vi "Reformat.vi"(5 "Pretty Print?":bool, 7 "error in (no error)":errorcluster, 8 "Offset":i32, 10 "JSON":string) -> (0 "error out":errorcluster, 1 "Offset after":i32, 3 "<JSON>":string)   [LabVIEW 2015, in "JSONtext.lvlib"]
doc: "Reformat a JSON Value, either packed with all unneeded whitespace removed, or \"pretty printed\" with extra whitespace and new lines to make the JSON more human readable. This will also searve to validate the JSON."
uses:
  JSONtext.lvlib
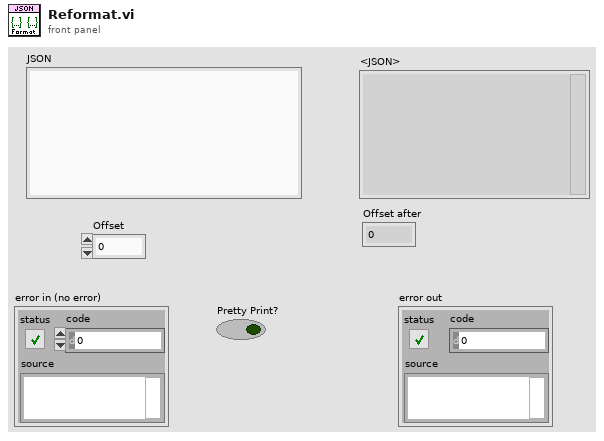
[diagram p1: front panel]
types:
  T1 = typedef "JSONtext.lvlib/Parsing State.ctl" = enum16{"Parser Error", "Object", "Array", "String", "Number/Other", "Leading Whitespace", "Object end", "Array end", "Value end"}
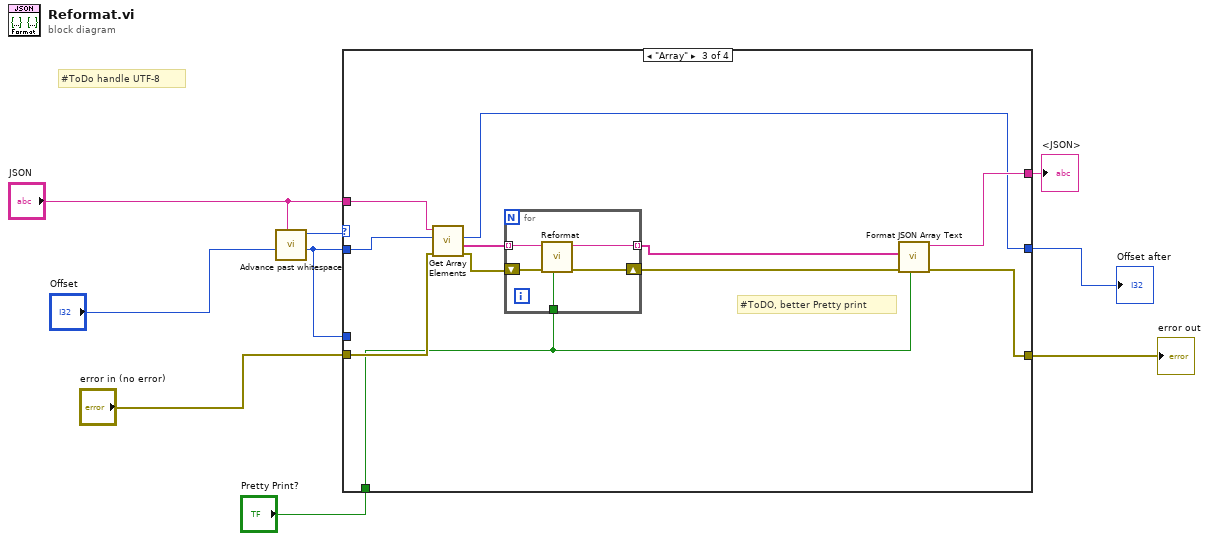
[diagram p0: block diagram]
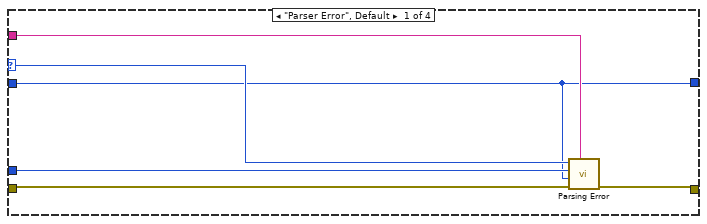
[diagram p2: hidden frame]
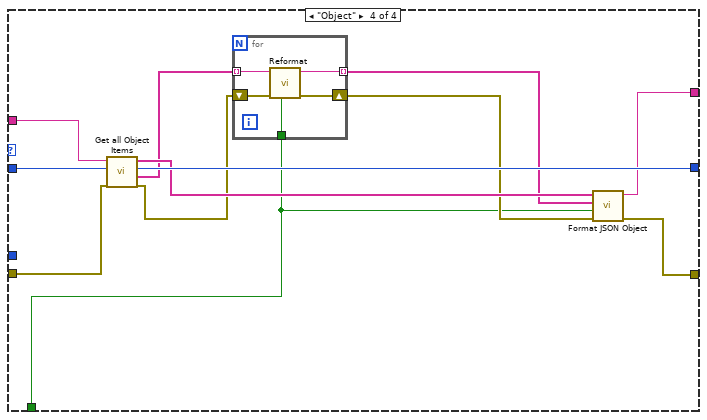
[diagram p4: hidden frame]
diagram:
  # "#ToDo handle UTF-8"
  n1 = call "Advance past whitespace.vi"("JSON"="JSON", "Offset"="Offset") -> ("Offset of first non-whitespace"=w2:i32, "Parser State"=w8:T1)  [unwired: 8 in]
  n2 = case shown="\"Array\"" w8 {
    selector: w8 -> [w13 _ _ _]
    tunnel: "JSON" -> [w11 w18 w29 w43]
    tunnel: w2 -> [w10 w16 w28 w46]
    tunnel: [w10 w16 w22 w45] -> w7
    tunnel: [_ w18 w26 w42] -> w5
    tunnel: [w15 w17 w24 w37] -> w4
    tunnel: "error in (no error)" -> [w14 w17 w23 w36]
    tunnel: w2 -> [w12 _ _ _]
    tunnel: "Pretty Print?" -> [_ _ w21 w35]
    frame "Parser Error", Default {
      n3 = call "Parsing Error.vi"("JSON"=w11, "error in (no error)"=w14, "Offset past match"=w10, "Value start"=w12, "State"=w13) -> ("error out"=w15:errorcluster)  [unwired: 6 in]
    }
    frame "String", "Number/Other" {
    }
    frame "Array" {
      # "#ToDO, better Pretty print"
      n4 = call "Get Array Elements.vi"("error in (no error)"=w23, "Offset"=w28, "JSON"=w29) -> ("error out"=w25:errorcluster, "<JSON>"=w27:string[], "Offset past Array"=w22:i32)  [unwired: 5 in, 1 out]
      n5 = for {
        tunnel: w27 -> [w34] mode=indexing
        tunnel: [w33] -> w20 mode=indexing
        shift-right: [w31] -> w19
        shift-left: w25 -> [w32]
        tunnel: w21 -> [w30]
        n6 = call "Reformat.vi"("Pretty Print?"=w30, "error in (no error)"=w32, "JSON"=w34) -> ("error out"=w31:errorcluster, "<JSON>"=w33:string)  [unwired: 5 in, 1 out]
      }
      n7 = call "Format JSON Array Text.vi"("Pretty Print?"=w21, "error in (no error)"=w19, "Array of JSON Text"=w20) -> ("error out"=w24:errorcluster, "<JSON>"=w26:string)  [unwired: 7 in]
    }
    frame "Object" {
      n8 = call "Get all Object Items.vi"("error in (no error)"=w36, "Offset"=w46, "JSON"=w43) -> ("error out"=w39:errorcluster, "<JSON>"=w41:string[], "Offset past Object"=w45:i32, "Names"=w44:string[])  [unwired: 5 in]
      n9 = for {
        tunnel: w41 -> [w51] mode=indexing
        tunnel: [w50] -> w40 mode=indexing
        shift-right: [w48] -> w38
        shift-left: w39 -> [w49]
        tunnel: w35 -> [w47]
        n10 = call "Reformat.vi"("Pretty Print?"=w47, "error in (no error)"=w49, "JSON"=w51) -> ("error out"=w48:errorcluster, "<JSON>"=w50:string)  [unwired: 5 in, 1 out]
      }
      n11 = call "Format JSON Object.vi"("error in (no error)"=w38, "Pretty Print?"=w35, "JSON elements"=w40, "Names"=w44) -> ("error out"=w37:errorcluster, "JSON Object Text out"=w42:string)  [unwired: 6 in]
    }
  }
  "Offset after" <- w7
  "<JSON>" <- w5
  "error out" <- w4
